vi "Py - CsB FL K.vi"(8 "error in":errorcluster, 9 "En":dbl, 10 "Lin":i32, 11 "Z":i32) -> (0 "error out":errorcluster, 3 "CsB FL K":dbl)   [LabVIEW 2023]
uses:
  global python version.vi
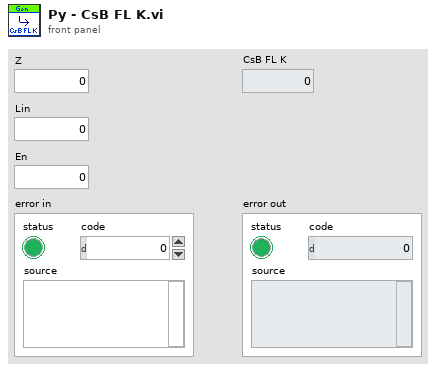
[diagram p1: front panel]
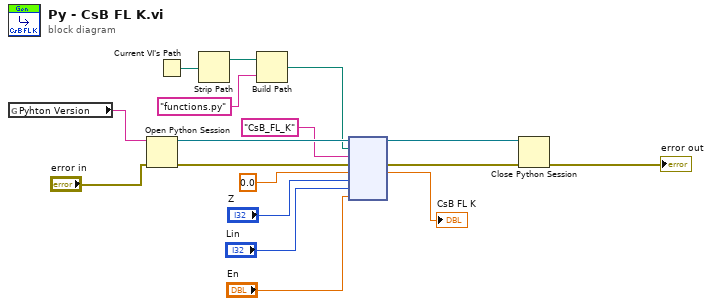
[diagram p0: block diagram]
diagram:
  n1 = global read "global python version.vi" "Pyhton Version"() -> (w5:string)
  n2 = Open Python Session(python version=w5, 3:"error in") -> (session out=w14:refnum<k35>, error out=w11:errorcluster)  [unwired: 1 in]
  n3 = Current VI's Path() -> (path=w16:path)
  n4 = Strip Path(path=w16) -> (stripped path=w15:path)  [unwired: 1 out]
  n5 = Build Path(base path=w15, name or relative path="functions.py") -> (appended path=w7:path)
  n6 = node(w14, w7, "CsB_FL_K", w11, 0.0, "Z", "Lin", "En") -> (w13:refnum<k35>, w12:errorcluster, →"CsB FL K":dbl)  [unwired: 3 in, 2 out]
  n7 = Close Python Session(session in=w13, error in=w12) -> (11:→"error out":errorcluster)
